vi "仁科空调状态解析.vi"(11 "系统参数输入":u16[](array[numeric])) -> (3 "运行状态":T1)   [LabVIEW 2016, in "环境动力监测库.lvlib" / "空调库.lvlib"]
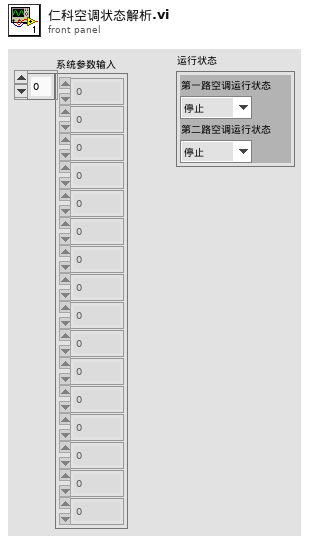
[diagram p1: front panel]
types:
  T1 = cluster{"第一路空调运行状态":enum16{"停止", "制冷", "制热", "未知"}, "第二路空调运行状态":enum16{"停止", "制冷", "制热", "未知"}}
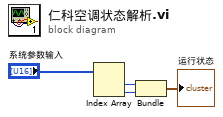
[diagram p0: block diagram]
diagram:
  n1 = Index Array(array="系统参数输入") -> (element #1=w3:u16, element #2=w2:u16)  [unwired: 2 in]
  n2 = Bundle(w3, w2) -> (→"运行状态":cluster{u16, u16})  [unwired: 1 in]
